vi "Get SMO Public API.vi"(8 "error in (no error)":errorcluster, 11 "Instrument.VRM In":refnum<class "Instrument.OxfordVRM.lvclass">) -> (0 "error out":errorcluster, 2 "Commands":string[](array[string]), 3 "Instrument.VRM out":refnum<class "Instrument.OxfordVRM.lvclass">)   [LabVIEW 2019, in "Instrument.OxfordVRM.lvclass"]
uses:
  Instrument.OxfordVRM.lvclass
  C:/Program Files/National Instruments/LabVIEW 2019/user.lib/LevyLab/Instrument Framework/Instrument/Instrument.lvclass
  Typedefs/Instrument.VRM.publicCommands-enum.ctl
  a30af0d3-6c03-4a39-9997-ffb264a7dac7.vi
  <vilib>/Utility/Data Type/Get Type Information.vi
  <vilib>/Utility/Data Type/Get Numeric Information.vi
  <userlib>/_OpenG.lib/lvdata/lvdata.llb/Unwrap VVariant__ogtk.vi
  <userlib>/LevyLab/Instrument Framework/Instrument Types/Cryostat/Instrument.Cryostat.lvclass
  <userlib>/LevyLab/Instrument Framework/Instrument/Instrument.lvclass
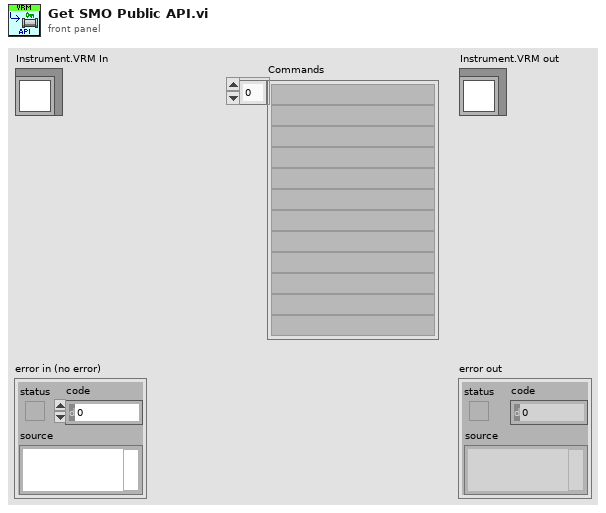
[diagram p1: front panel]
types:
  T1 = typedef "Instrument.OxfordVRM.lvclass/Instrument.VRM.publicCommands-enum.ctl" = enum16{"setMagnet", "setMagnetVector", "getMagnet", "getMagnetVector", "getMagnetTarget", "getMagnetVectorTarget"}
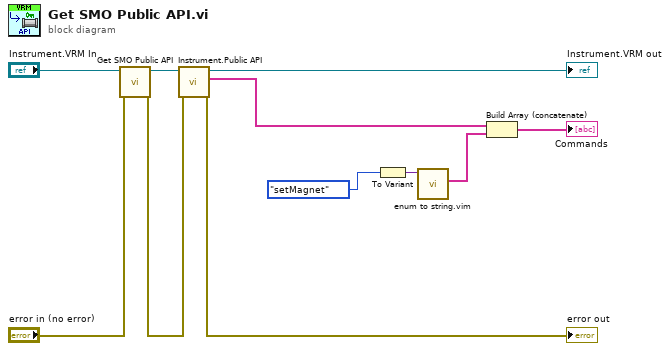
[diagram p0: block diagram]
diagram:
  n1 = call-parent "Get SMO Public API.vi"("error in (no error)"="error in (no error)", "Instrument.Cryostat in"="Instrument.VRM In") -> ("error out"=w2:errorcluster, "Instrument.Cryostat out"=w4:refnum<class "Instrument.OxfordVRM.lvclass">)  [unwired: 7 in, 1 out]
  n2 = call <userlib>:"Instrument.Public API.vi"("error in (no error)"=w2, "Instrument in"=w4) -> ("error out"=→"error out":errorcluster, "commands (this level)"=w6:string[], "Instrument out"=→"Instrument.VRM out":refnum<class "Instrument.OxfordVRM.lvclass">)  [unwired: 7 in]
  n3 = To Variant(anything=Instrument.VRM.publicCommands-enum."setMagnet" ("Commands")) -> (Variant=w9:variant)
  n4 = call "enum to string.vim"("enum in"=w9) -> ("strings out"=w7:string[])  [unwired: 9 in, 1 out]
  n5 = Build Array (concatenate)(w6, w7) -> (→"Commands":string[])
